vi "AI Level Trigger.vi"(10 "Trigger Level":i16, 11 "Data In":u32) -> (3 "Trigger":bool)   [LabVIEW 2010]
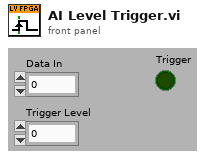
[diagram p1: front panel]
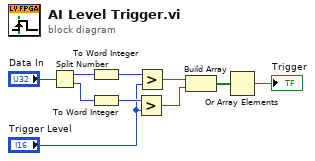
[diagram p0: block diagram]
diagram:
  n1 = Split Number(x="Data In") -> (hi(x)=w6:u16, lo(x)=w8:u16)
  n2 = To Word Integer(number=w6) -> (16bit integer=w5:i16)
  n3 = To Word Integer(number=w8) -> (16bit integer=w7:i16)
  n4 = Greater?(x=w7, y="Trigger Level") -> (0:w2:bool)
  n5 = Greater?(x=w5, y="Trigger Level") -> (0:w3:bool)
  n6 = Build Array(w3, w2) -> (w1:bool[])
  n7 = Or Array Elements(Boolean array=w1) -> (logical OR=→"Trigger":bool)
